vi "mlProject_testCNet.vi"() -> ()   [LabVIEW 2016]
uses:
  <vilib>/Analysis/2dsp.llb/2D Convolution (DBL).vi
  CNetLib/CNet.lvlib
  <vilib>/Analysis/Matrix/NI_Matrix.lvlib
  <vilib>/Analysis/NI_AALBase.lvlib
  <vilib>/Analysis/NI_AALPro.lvlib
  <vilib>/Analysis/7linalg.llb/Real Matrix Exp.vi
  <vilib>/Analysis/Matrix/Numeric/Conversions/Array To Matrix - RA2.vi
  <vilib>/Analysis/Matrix/Numeric/Conversions/Matrix To Array - RM.vi
panel:
  out "cols out":u32
  out "rows out":u32
  in  "CNet path":path
  out "Time [ms]":dbl
  in  "stop 2":bool
  out "C++ Address":i64
  out "size(s)":i32[](array[numeric])
  in  "Load from file":bool
  in  "adam":bool
  in  "weight_normalization":bool
  in  "batch_update":u32=3
  out "layer weights":sgl[][](graph)
  in  "Conjugate":bool
  in  "save to file":bool
  out "layerNumber":u32
  out "actual output":dbl[][](graph)
  out "Error":sgl[](graph)
  in  "eta":sgl=0.0001
  out "error":sgl
  in  "Validate":bool
  out "output Prediction":dbl[][](graph)
  out "Runs":i32
  in  "milliseconds to wait":u32=10
  in  "stop":bool
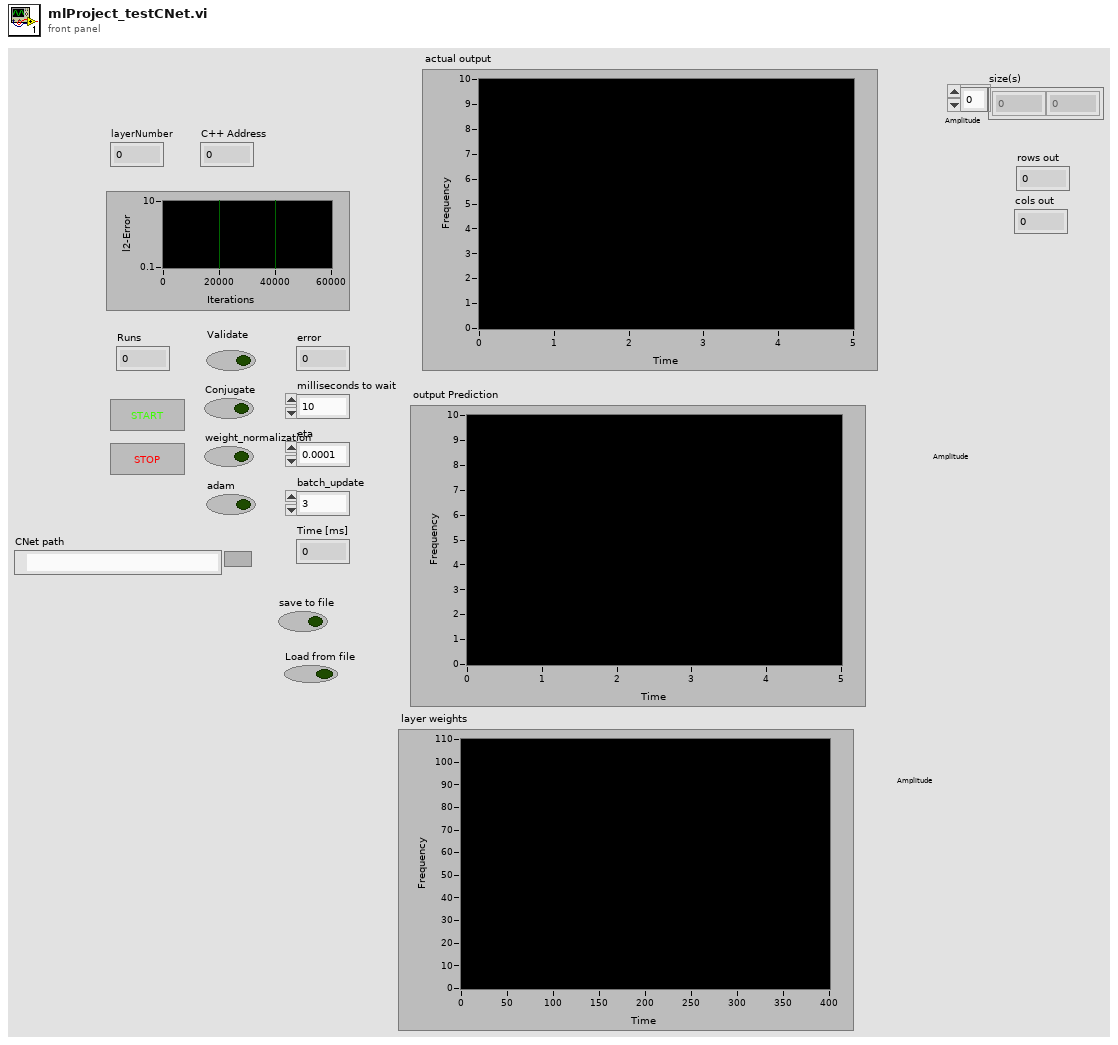
[diagram p1: front panel]
types:
  T1 = typedef "NI_Matrix.lvlib/RealMatrix.ctl" = dbl[][]
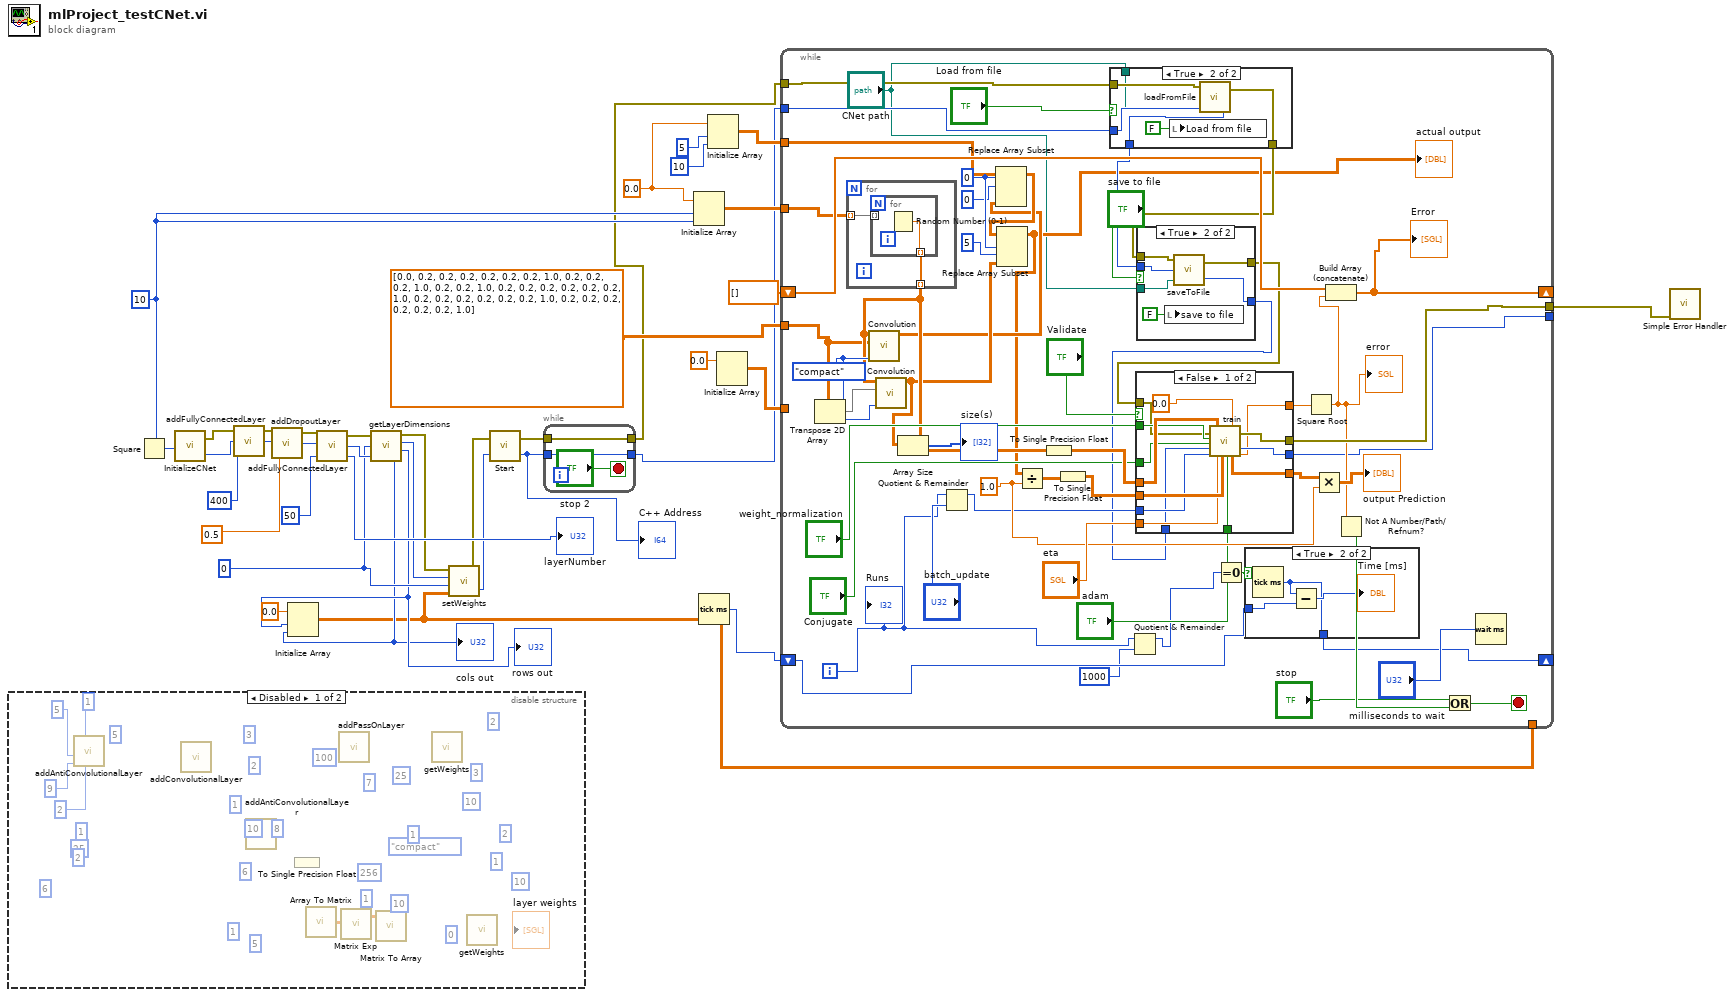
[diagram p0: block diagram]
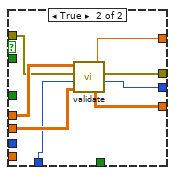
[diagram p5: hidden frame]
diagram:
  w10 = u32 0 ("layer")
  w31 = 0.0 ("element")
  w33 = u32 10 ("NIN")
  n1 = disable-structure shown="Disabled" {
    frame Disabled {
      (unwired) u32 0 ("layer")
      w39 = u32 6 ("kernelXY")
      (unwired) u32 5 ("NOUTXY")
      (unwired) u32 1 ("stride")
      (unwired) u32 2 ("features")
      w40 = u32 25 ("NOUT")
      (unwired) u32 1 ("stride")
      w50 = u32 6 ("kernelXY")
      w49 = u32 5 ("kernelXY")
      (unwired) 1
      (unwired) u32 2 ("stride")
      (unwired) u32 2 ("kernelXY")
      w51 = u32 10 ("NOUTXY")
      (unwired) u32 25 ("NOUT")
      w53 = u32 8 ("kernelXY")
      w52 = u32 2 ("stride")
      (unwired) enum32{"full", "size X", "compact"}."compact" ("output size")
      (unwired) u32 100 ("NOUT")
      (unwired) u32 10 ("NOUTXY")
      (unwired) u32 3 ("kernelXY")
      (unwired) u32 1 ("stride")
      (unwired) u32 10 ("NOUTXY")
      (unwired) u32 3 ("kernelXY")
      (unwired) u32 1 ("stride")
      (unwired) u32 10 ("NOUTXY")
      w56 = u32 1 ("stride")
      (unwired) u32 7 ("kernelXY")
      (unwired) u32 256 ("NOUTXY")
      n2 = call "addAntiConvolutionalLayer.vi"("stride"=u32 1, "kernelXY"=u32 5, "features"=u32 2, "NOUTXY"=u32 9) -> ("error in (no error)"=w42:errorcluster, "ptr"=w43:i64, "error out"=w41:errorcluster, "ptr out"=w44:i64)  [unwired: 1 out]
      n3 = call "addConvolutionalLayer.vi"() -> ()  [unwired: 6 in, 3 out]
      n4 = call "addAntiConvolutionalLayer.vi"() -> ()  [unwired: 5 in, 3 out]
      n5 = To Single Precision Float() -> ()  [unwired: 1 in, 1 out]
      n6 = call-poly <vilib>:"Array To Matrix.vi"() -> ("Real Matrix"=w54:T1)  [unwired: 1 in]
      n7 = call "addPassOnLayer.vi"() -> ()  [unwired: 2 in, 3 out]
      n8 = call-poly <vilib>:"Matrix Exp.vi"("Input Matrix"=w54) -> ("Matrix Exp"=w55:T1)  [unwired: 1 in, 1 out]
      n9 = call-poly <vilib>:"Matrix To Array.vi"("Real Matrix"=w55) -> ()  [unwired: 1 out]
      n10 = call "getWeights.vi"() -> ()  [unwired: 4 in, 3 out]
      n11 = call "getWeights.vi"() -> ()  [unwired: 4 in, 3 out]
    }
    frame Enabled {
    }
  }
  n12 = Square(x=w33) -> (x^2=w32:u32)
  n13 = call "InitializeCNet.vi"("NIN"=w32) -> ("ptr"=w20:i64, "error out"=w21:errorcluster)  [unwired: 1 in]
  n14 = call "addFullyConnectedLayer.vi"("NOUT"=u32 400, "ptr"=w20, "error in (no error)"=w21) -> ("ptr out"=w3:i64, "error out"=w5:errorcluster)  [unwired: 1 out]
  n15 = call "addDropoutLayer.vi"("ratio set zero"=sgl 0.5 ("ratio"), "ptr"=w3, "error in (no error)"=w5) -> ("ptr out"=w2:i64, "error out"=w4:errorcluster)  [unwired: 1 out]
  n16 = call "addFullyConnectedLayer.vi"("NOUT"=u32 50, "ptr"=w2, "error in (no error)"=w4) -> ("layers"=→"layerNumber":u32, "ptr out"=w15:i64, "error out"=w17:errorcluster)
  n17 = call "getLayerDimensions.vi"("error in (no error)"=w17, "layer"=w10, "ptr"=w15) -> ("error out"=w14:errorcluster, "ptr out"=w12:i64, "rows out"=w9:u32, "cols out"=w8:u32)
  "rows out" <- w9
  "cols out" <- w8
  n18 = Initialize Array(sgl 0.0 ("element"), w9, w8) -> (w6:sgl[][])
  n19 = call "setWeights.vi"("weights"=w6, "layer"=w10, "ptr"=w12, "error in (no error)"=w14) -> ("ptr out"=w11:i64, "error out"=w13:errorcluster)
  n20 = call "Start.vi"("ptr"=w11, "error in (no error)"=w13) -> ("ptr out"=w24:i64, "error out"=w26:errorcluster)
  "C++ Address" <- w24
  n21 = while {
    tunnel: w26 -> [w59]
    tunnel: w24 -> [w58]
    tunnel: [w59] -> w23
    tunnel: [w58] -> w25
    stop <- "stop 2" stop-if-true
  }
  n22 = Initialize Array(w31, w33, w33) -> (w34:dbl[][])
  n23 = Tick Count (ms)() -> (millisecond timer value=w18:u32)
  n24 = Initialize Array(w31, 5 ("dimension size"), 10 ("dimension size")) -> (w28:dbl[][])
  n25 = Initialize Array(sgl 0.0 ("element")) -> (w37:sgl[][])  [unwired: 2 in]
  n26 = while {
    tunnel: w37 -> [_]
    tunnel: w23 -> [w91]
    tunnel: [w85] -> w22
    shift-right: [w107] -> _
    shift-left: sgl[] [] -> [w108]
    tunnel: w25 -> [w89]
    tunnel: [w61] -> _
    tunnel: dbl[][] [[0.0, 0.2, 0.2, 0.2, 0.2, 0.2], [0.2, 1.0, 0.2, 0.2, 0.2, 1.0], [0.2, 0.2, 1.0, 0.2, 0.2, 0.2], [0.2, 0.2, 0.2, 1.0, 0.2, 0.2], [0.2, 0.2, 0.2, 0.2, 1.0, 0.2], [0.2, 0.2, 0.2, 0.2, 0.2, 1.0]] -> [w75]
    tunnel: w34 -> [w99]
    tunnel: w28 -> [w81]
    shift-right: [w63] -> _
    shift-left: w18 -> [w64]
    tunnel: w6 -> [_]
    i -> [w67]
    stop <- w69 stop-if-true
    w80 = 0 ("disabled index (col)")
    w84 = enum32{"full", "size X", "compact"}."compact" ("output size")
    w102 = 1.0 ("element")
    n27 = Transpose 2D Array(2D array=w75) -> (transposed array=w74:dbl[][])
    n28 = for {
      tunnel: w99 -> [w125] mode=indexing
      tunnel: [w124] -> w83 mode=indexing
      n29 = for {
        tunnel: w125 -> [_] mode=indexing
        tunnel: [w126] -> w124 mode=indexing
        n30 = Random Number (0-1)() -> (number: 0 to 1=w126:dbl)
      }
    }
    n31 = call-poly <vilib>:"Convolution.vi"("output size"=w84, "Y"=w75, "X"=w83) -> ("X * Y"=w73:dbl[][])  [unwired: 7 in, 1 out]
    n32 = call-poly <vilib>:"Convolution.vi"("output size"=w84, "Y"=w74, "X"=w83) -> ("X * Y"=w78:dbl[][])  [unwired: 7 in, 1 out]
    n33 = Array Size(array=w78) -> (size(s)=→"size(s)":i32[])
    n34 = Quotient & Remainder(x=w67, y="batch_update") -> (x-y*floor(x/y)=w97:u32)  [unwired: 1 out]
    n35 = Replace Array Subset(array=w81, new element=w73, index (row)=0, index (col)=w80) -> (w76:dbl[][])
    n36 = Replace Array Subset(array=w76, new element=w78, index (row)=w80, index (col)=5 ("index (row)")) -> (w68:dbl[][])
    "actual output" <- w68
    n37 = Divide(x=w68, y=w102) -> (x/y=w101:dbl[][])
    n38 = To Single Precision Float(number=w83) -> (single precision float=w95:sgl[][])
    n39 = To Single Precision Float(number=w101) -> (single precision float=w100:sgl[][])
    n40 = case shown="True" "Load from file" {
      tunnel: w91 -> [w117 w122]
      tunnel: [w117 w121] -> w90
      tunnel: w89 -> [w116 w120]
      tunnel: [w116 w119] -> w88
      tunnel: "CNet path" -> [_ w118]
      frame False {
      }
      frame True {
        n41 = local write "Load from file"(FALSE ("Load from file")) -> ()
        n42 = call "loadFromFile.vi"("path"=w118, "ptr"=w120, "error in (no error)"=w122) -> ("ptr out"=w119:i64, "error out"=w121:errorcluster)
      }
    }
    n43 = Quotient & Remainder(x=w67, y=1000) -> (x-y*floor(x/y)=w65:i32)  [unwired: 1 out]
    n44 = case shown="True" "save to file" {
      tunnel: w90 -> [w128 w132]
      tunnel: [w128 w131] -> w86
      tunnel: w88 -> [w127 w133]
      tunnel: [w127 w130] -> w87
      tunnel: "CNet path" -> [_ w129]
      frame False {
      }
      frame True {
        n45 = local write "save to file"(FALSE ("save to file")) -> ()
        n46 = call "saveToFile.vi"("path"=w129, "ptr"=w133, "error in (no error)"=w132) -> ("ptr out"=w130:i64, "error out"=w131:errorcluster)
      }
    }
    n47 = case shown="False" "Validate" {
      tunnel: [w148 w156] -> w85
      tunnel: [w145 w153] -> w104
      tunnel: w95 -> [w147 w151]
      tunnel: [w141 w155] -> w106
      tunnel: w100 -> [w146 w154]
      tunnel: "eta" -> [w144 _]
      tunnel: [w142 w152] -> w61
      tunnel: w86 -> [w138 w150]
      tunnel: w97 -> [w140 _]
      tunnel: "weight_normalization" -> [w139 _]
      tunnel: "Conjugate" -> [w137 _]
      tunnel: w87 -> [w136 w149]
      tunnel: "adam" -> [w135 _]
      frame False {
        n48 = call "train.vi"("error in (no error)"=w138, "weight_normalization"=w139, "Conjugate"=w137, "ptr"=w136, "batch_update"=w140, "input"=w147, "eta"=w144, "outputDesired"=w146, "adam"=w135, "lambda"=sgl 0.0) -> ("prediction"=w145:sgl[][], "error out"=w148:errorcluster, "ptr out"=w142:i64, "error"=w141:sgl)  [unwired: 6 in]
      }
      frame True {
        n49 = call "validate.vi"("output"=w154, "ptr"=w149, "error in (no error)"=w150, "input"=w151) -> ("prediction"=w153:sgl[][], "ptr out"=w152:i64, "error out"=w156:errorcluster, "error"=w155:sgl)
      }
    }
    n50 = Equal To 0?(x=w65) -> (x = 0?=w66:bool)
    n51 = case shown="True" w66 {
      tunnel: w64 -> [w112 w115]
      tunnel: [w112 w113] -> w63
      frame False {
      }
      frame True {
        n52 = Tick Count (ms)() -> (millisecond timer value=w113:u32)
        n53 = Subtract(x=w113, y=w115) -> (x-y=→"Time [ms]":u32)
      }
    }
    n54 = Square Root(x=w106) -> (sqrt(x)=w72:sgl)
    "error" <- w72
    n55 = Multiply(x=w104, y=w102) -> (x*y=→"output Prediction":dbl[][])
    n56 = Build Array (concatenate)(w108, w72) -> (w107:sgl[])
    "Error" <- w107
    n57 = Not A Number/Path/Refnum?(number/path/refnum=w72) -> (NaN/Path/Refnum?=w71:bool)
    n58 = Or(x="stop", y=w71) -> (x .or. y?=w69:bool)
    n59 = Wait (ms)(milliseconds to wait="milliseconds to wait") -> ()  [unwired: 1 out]
    "Runs" <- w67
  }
  n60 = call <vilib>:"Simple Error Handler.vi"("error in (no error)"=w22) -> ()  [unwired: 4 in, 5 out]
